vi "Publish Data to Array.vi"(10 "Group Results By":T1, 11 "Publish Data":T2[](array[typedef])) -> (2 "Status Color":u32[](array[numeric]), 3 "Data[]":string[][](array[string]))   [LabVIEW 2019, in "STS_LTRV.lvlib"]
uses:
  STS_LTRV.lvlib
  TypeDefs/UI Data.ctl
  TypeDefs/Publish Data.ctl
  TypeDefs/NumericLimit Data.ctl
  TypeDefs/Group Results By.ctl
  d5af9614-e442-42f0-86bd-407a04029839.vi
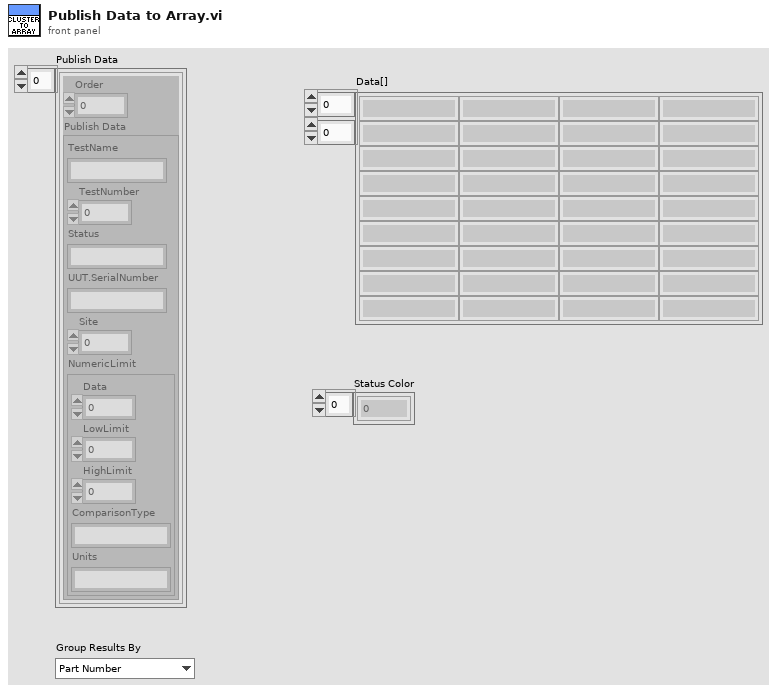
[diagram p1: front panel]
types:
  T1 = typedef "STS_LTRV.lvlib/Group Results By.ctl" = enum16{"Part Number", "Test Number"}
  T2 = typedef "STS_LTRV.lvlib/UI Data.ctl" = cluster{"Order":u64, "Publish Data":T3}
  T3 = typedef "STS_LTRV.lvlib/Publish Data.ctl" = cluster{"TestName":string, "TestNumber":dbl, "Status":string, "UUT.SerialNumber":string, "Site":dbl, "NumericLimit":T4}
  T4 = typedef "STS_LTRV.lvlib/NumericLimit Data.ctl" = cluster{"Data":dbl, "LowLimit":dbl, "HighLimit":dbl, "ComparisonType":string, "Units":string}
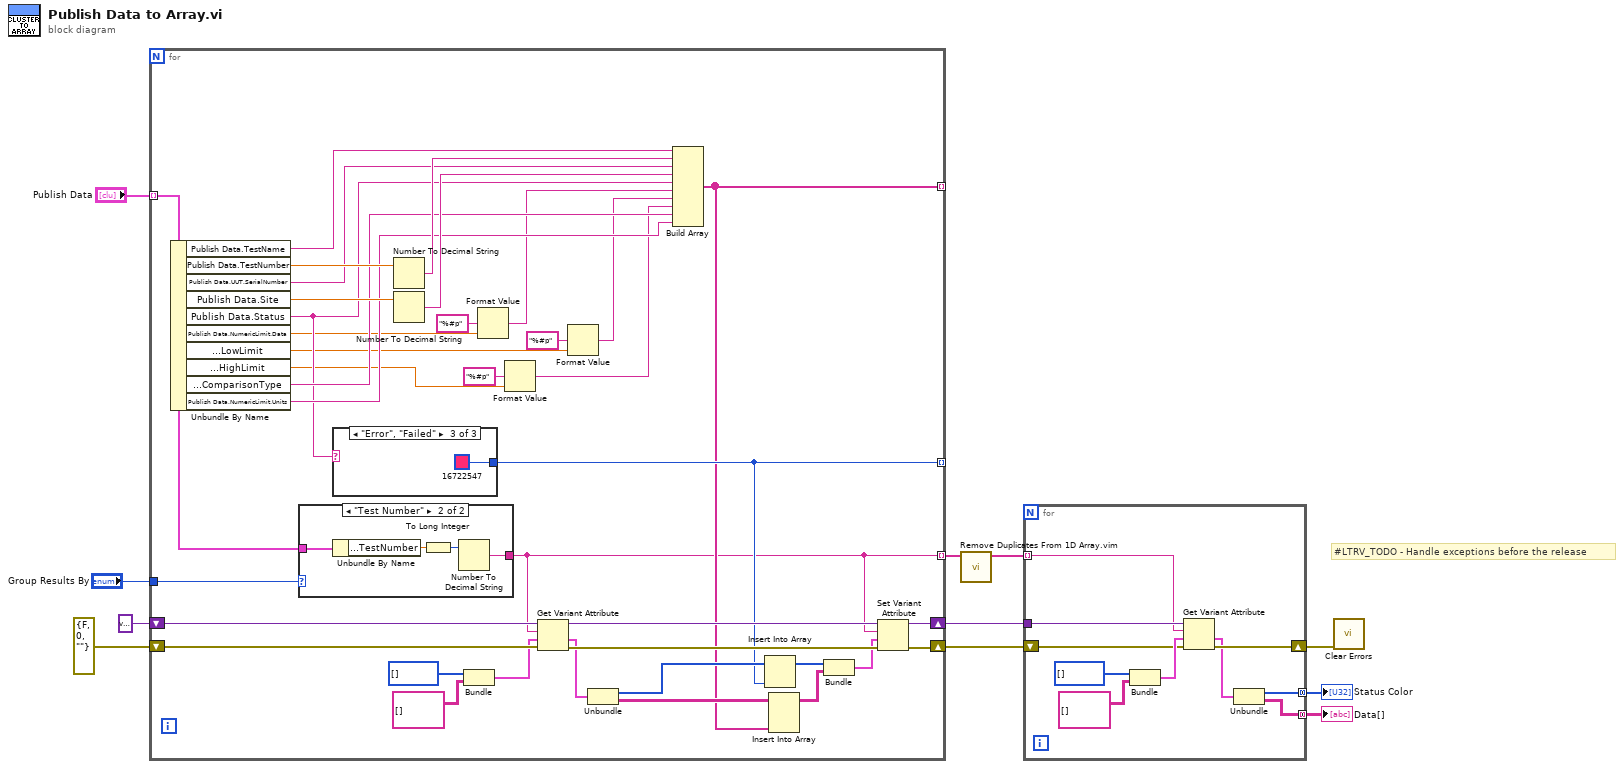
[diagram p0: block diagram]
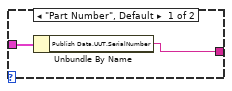
[diagram p2: hidden frame]
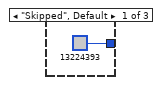
[diagram p3: hidden frame]
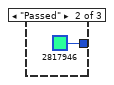
[diagram p4: hidden frame]
diagram:
  # "#LTRV_TODO - Handle exceptions before the release"
  n1 = for {
    tunnel: [w16] -> _ mode=indexing
    tunnel: "Publish Data" -> [w28] mode=indexing
    tunnel: [w18] -> _ mode=indexing
    tunnel: "Group Results By" -> [w29]
    shift-right: [w21] -> w5
    shift-left: variant -> [w31]
    shift-right: [w22] -> w6
    shift-left: errorcluster {"status"=FALSE, "code"=0, "source"=""} ("error in") -> [w30]
    tunnel: [w12] -> w7 mode=indexing
    n2 = Unbundle By Name(w28) -> ("Publish Data.TestName"=w47:string, "Publish Data.TestNumber"=w49:dbl, "Publish Data.UUT.SerialNumber"=w45:string, "Publish Data.Site"=w48:dbl, "Publish Data.Status"=w41:string, "Publish Data.NumericLimit.Data"=w40:dbl, "Publish Data.NumericLimit.LowLimit"=w36:dbl, "Publish Data.NumericLimit.HighLimit"=w33:dbl, "Publish Data.NumericLimit.ComparisonType"=w43:string, "Publish Data.NumericLimit.Units"=w42:string)
    n3 = case shown="\"Test Number\"" w29 {
      tunnel: w28 -> [w51 w55]
      tunnel: [w50 w52] -> w12
      frame "Part Number", Default {
        n4 = Unbundle By Name(w51) -> ("Publish Data.UUT.SerialNumber"=w50:string)
      }
      frame "Test Number" {
        n5 = Unbundle By Name(w55) -> ("Publish Data.TestNumber"=w54:dbl)
        n6 = To Long Integer(number=w54) -> (32bit integer=w53:i32)
        n7 = Number To Decimal String(number=w53) -> (decimal integer string=w52:string)  [unwired: 1 in]
      }
    }
    n8 = case shown="\"Error\", \"Failed\"" w41 {
      tunnel: [u32 13224393 u32 2817946 u32 16722547] -> w18
      frame "Skipped", Default {
      }
      frame "Passed" {
      }
      frame "Error", "Failed" {
      }
    }
    n9 = Number To Decimal String(number=w49) -> (decimal integer string=w46:string)  [unwired: 1 in]
    n10 = Number To Decimal String(number=w48) -> (decimal integer string=w44:string)  [unwired: 1 in]
    n11 = Bundle(u32[] [], "appended array"=string[][] []) -> (w25:cluster{u32[], "appended array":string[][]})  [unwired: 1 in]
    n12 = Format Value(format string="%#p", value (0)=w40) -> (output string=w39:string)  [unwired: 1 in]
    n13 = Format Value(format string="%#p", value (0)=w33) -> (output string=w32:string)  [unwired: 1 in]
    n14 = Get Variant Attribute(Variant=w31, name=w12, default value (empty Variant)=w25, error in=w30) -> (duplicate Variant=w23:variant, value=w20:cluster{u32[], "appended array":string[][]}, error out=w24:errorcluster)  [unwired: 1 out]
    n15 = Format Value(format string="%#p", value (0)=w36) -> (output string=w35:string)  [unwired: 1 in]
    n16 = Unbundle(w20) -> (w19:u32[], "appended array"=w17:string[][])
    n17 = Build Array(w47, w46, w45, w44, w41, w39, w35, w32, w43, w42) -> (w16:string[])
    n18 = Insert Into Array(array=w19, new element=w18) -> (w15:u32[])  [unwired: 1 in]
    n19 = Insert Into Array(array=w17, new element=w16) -> (w14:string[][])  [unwired: 2 in]
    n20 = Bundle(w15, "appended array"=w14) -> (w13:cluster{u32[], "appended array":string[][]})  [unwired: 1 in]
    n21 = Set Variant Attribute(Variant=w23, name=w12, value=w13, error in=w24) -> (Variant out=w21:variant, error out=w22:errorcluster)  [unwired: 1 out]
  }
  n22 = call "Remove Duplicates From 1D Array.vim"("array"=w7) -> ("array with duplicates removed"=w4:string[])  [unwired: 10 in]
  n23 = for {
    tunnel: w5 -> [w64]
    tunnel: w4 -> [w63] mode=indexing
    shift-right: [w62] -> w1
    shift-left: w6 -> [w65]
    tunnel: [w60] -> w2 mode=concatenating
    tunnel: [w59] -> w3 mode=concatenating
    n24 = Bundle(u32[] [], "appended array"=string[][] []) -> (w68:cluster{u32[], "appended array":string[][]})  [unwired: 1 in]
    n25 = Get Variant Attribute(Variant=w64, name=w63, default value (empty Variant)=w68, error in=w65) -> (value=w61:cluster{u32[], "appended array":string[][]}, error out=w62:errorcluster)  [unwired: 2 out]
    n26 = Unbundle(w61) -> (w60:u32[], "appended array"=w59:string[][])
  }
  "Data[]" <- w3
  "Status Color" <- w2
  n27 = call <vilib>:"Clear Errors.vi"("error in (no error)"=w1) -> ()  [unwired: 5 in, 2 out]
